vi "PathPlanner_PathFinding_EnsureInitialized.vi"(8 "error in (no error)":errorcluster) -> (0 "error out":errorcluster)   [LabVIEW 2019, in "PathPlanner24.lvlib"]
uses:
  PathPlanner_PathFinder_Globals.vi
  PathPlanner24.lvlib
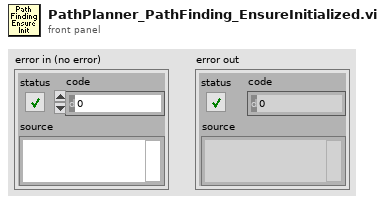
[diagram p1: front panel]
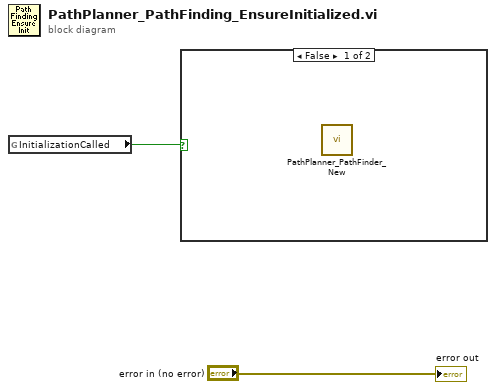
[diagram p0: block diagram]
diagram:
  n1 = global read "PathPlanner_PathFinder_Globals.vi" "InitializationCalled"() -> (w1:bool)
  n2 = case shown="False" w1 {
    frame False {
      n3 = call "PathPlanner_PathFinder_New.vi"() -> ()  [unwired: 11 in, 1 out]
    }
    frame True {
    }
  }
  "error out" <- "error in (no error)"
